vi "RM-set-command.vi"(8 "error in (no error)":errorcluster, 9 "command":T1={"type"=enum."abs_move", "position"=10.0, "velocity"=100.0, "acc"=3000.0, "dec"=3000.0, "band"=0.1, "push force"=30.0, "push distance"=30.0, "delay time"=500, "next command index"=-1}, 10 "command index":u16, 11 "MB_Master_Serial输入":refnum<class "MB_Master_Serial.lvclass">) -> (0 "error out":errorcluster, 3 "MB_Master_Serial输出":refnum<class "MB_Master_Serial.lvclass">)   [LabVIEW 2014]
uses:
  <vilib>/Plasmionique/MB Master/MB_Master_Serial/MB_Master_Serial.lvclass
  <vilib>/Plasmionique/MB Master/MB Master.lvlib
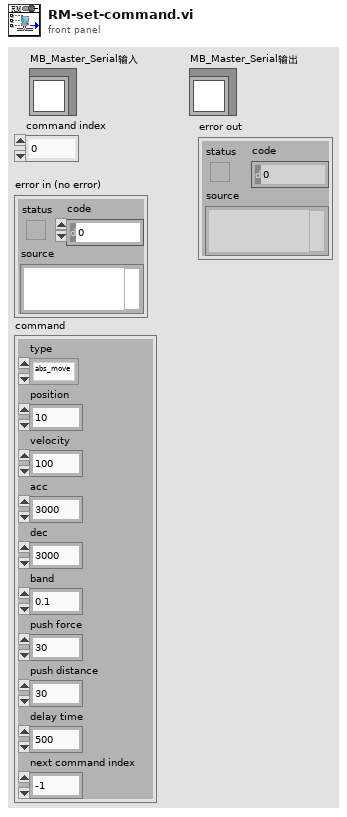
[diagram p1: front panel]
types:
  T1 = cluster{"type":enum16{"none", "go_home", "delay", "abs_move", "push", "inc_move"}, "position":dbl, "velocity":dbl, "acc":dbl, "dec":dbl, "band":dbl, "push force":dbl, "push distance":dbl, "delay time":i32, "next command index":i32}
  T2 = enum16{"none", "go_home", "delay", "abs_move", "push", "inc_move"}
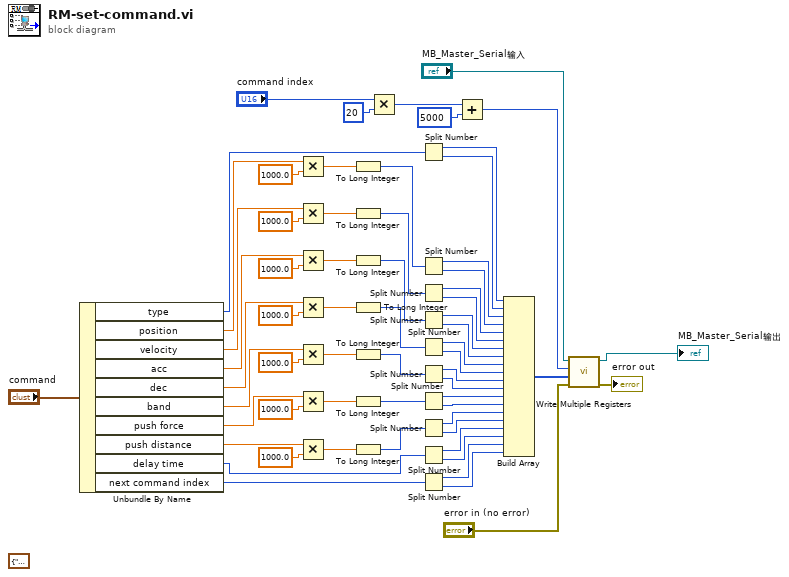
[diagram p0: block diagram]
diagram:
  (unwired) T1 {"type"=enum."abs_move", "position"=10.0, "velocity"=100.0, "acc"=3000.0, "dec"=3000.0, "band"=0.1, "push force"=30.0, "push distance"=30.0, "delay time"=500, "next command index"=-1}
  n1 = Unbundle By Name("command") -> ("type"=w54:T2, "position"=w53:dbl, "velocity"=w38:dbl, "acc"=w37:dbl, "dec"=w36:dbl, "band"=w20:dbl, "push force"=w19:dbl, "push distance"=w18:dbl, "delay time"=w9:i32, "next command index"=w6:i32)
  n2 = Multiply(x=w53, y=1000.0) -> (x*y=w51:dbl)
  n3 = Multiply(x=w38, y=1000.0) -> (x*y=w46:dbl)
  n4 = Multiply(x=w37, y=1000.0) -> (x*y=w43:dbl)
  n5 = Multiply(x=w36, y=1000.0) -> (x*y=w40:dbl)
  n6 = Multiply(x=w20, y=1000.0) -> (x*y=w28:dbl)
  n7 = Multiply(x=w19, y=1000.0) -> (x*y=w25:dbl)
  n8 = Multiply(x=w18, y=1000.0) -> (x*y=w22:dbl)
  n9 = To Long Integer(number=w51) -> (32bit integer=w50:i32)
  n10 = To Long Integer(number=w46) -> (32bit integer=w45:i32)
  n11 = To Long Integer(number=w43) -> (32bit integer=w42:i32)
  n12 = To Long Integer(number=w40) -> (32bit integer=w39:i32)
  n13 = To Long Integer(number=w28) -> (32bit integer=w27:i32)
  n14 = To Long Integer(number=w25) -> (32bit integer=w24:i32)
  n15 = To Long Integer(number=w22) -> (32bit integer=w21:i32)
  n16 = Multiply(x="command index", y=u16 20) -> (x*y=w3:u16)
  n17 = Split Number(x=w54) -> (hi(x)=w59:u8, lo(x)=w60:u8)
  n18 = Split Number(x=w50) -> (hi(x)=w49:u16, lo(x)=w48:u16)
  n19 = Split Number(x=w45) -> (hi(x)=w35:u16, lo(x)=w34:u16)
  n20 = Split Number(x=w42) -> (hi(x)=w33:u16, lo(x)=w32:u16)
  n21 = Split Number(x=w39) -> (hi(x)=w31:u16, lo(x)=w30:u16)
  n22 = Split Number(x=w27) -> (hi(x)=w17:u16, lo(x)=w16:u16)
  n23 = Split Number(x=w24) -> (hi(x)=w15:u16, lo(x)=w14:u16)
  n24 = Split Number(x=w21) -> (hi(x)=w13:u16, lo(x)=w12:u16)
  n25 = Split Number(x=w9) -> (hi(x)=w11:u16, lo(x)=w10:u16)
  n26 = Split Number(x=w6) -> (hi(x)=w8:u16, lo(x)=w7:u16)
  n27 = Add(x=w3, y=u16 5000 ("starting address")) -> (x+y=w1:u16)
  n28 = Build Array(w59, w60, w49, w48, w35, w34, w33, w32, w31, w30, w17, w16, w15, w14, w13, w12, w11, w10, w8, w7) -> (w58:u16[])
  n29 = call <vilib>:"Write Multiple Registers.vi"("error in (no error)"="error in (no error)", "values"=w58, "starting address"=w1, "MB session in"="MB_Master_Serial输入") -> ("error out"=→"error out":errorcluster, "MB session out"=→"MB_Master_Serial输出":refnum<class "MB_Master_Serial.lvclass">)  [unwired: 6 in]
